vi "Init Msg Input.vi"(6 "Teller":refnum<class "Teller.lvclass">) -> (2 "Msg Input":refnum<class "Msg Input.lvclass">)   [LabVIEW 2020, in "jettl.lvlib" / "Stopping jettl Msg.lvlib" / "Stopping Msg Input.lvlib"]
doc: "jettl 6.12.1.94\nNathan Davis - Nathan Davis\nCopyright (c) 2026, Nathan Davis\nMIT"
uses:
  Stopping Msg Input.lvlib
  Msg Input/Msg Input.lvclass
  Teller/Teller.lvclass
  Stopping Msg Input/Stopping Msg Input.lvclass
  C:/git/jettl/src/jettl/jettl/Msg Input/Msg Input.lvclass
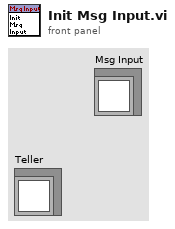
[diagram p1: front panel]
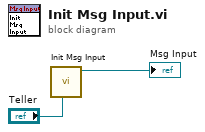
[diagram p0: block diagram]
diagram:
  n1 = call "Init Msg Input.vi"("Teller"="Teller") -> ("Stopping Msg Input out"=→"Msg Input":refnum<class "Stopping Msg Input.lvclass">)  [unwired: 10 in]
